vi "Get All Components From Config Browser.vi"() -> (2 "UniqueIDs":string[](array[string]), 3 "Names":string[](array[string]), 5 "error out":errorcluster)   [LabVIEW 2009]
doc: "Gets a list of all configured Horiba Jobin Yvon devices from the computer's registry"
panel:
  in  "error in (no error)":errorcluster
  in  "Config Browser":refnum<k7>
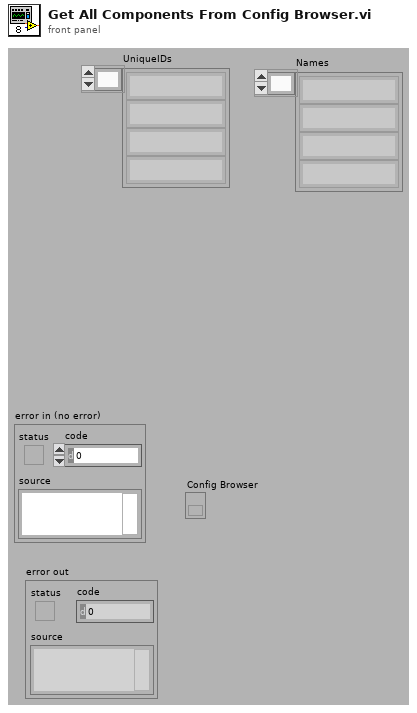
[diagram p1: front panel]
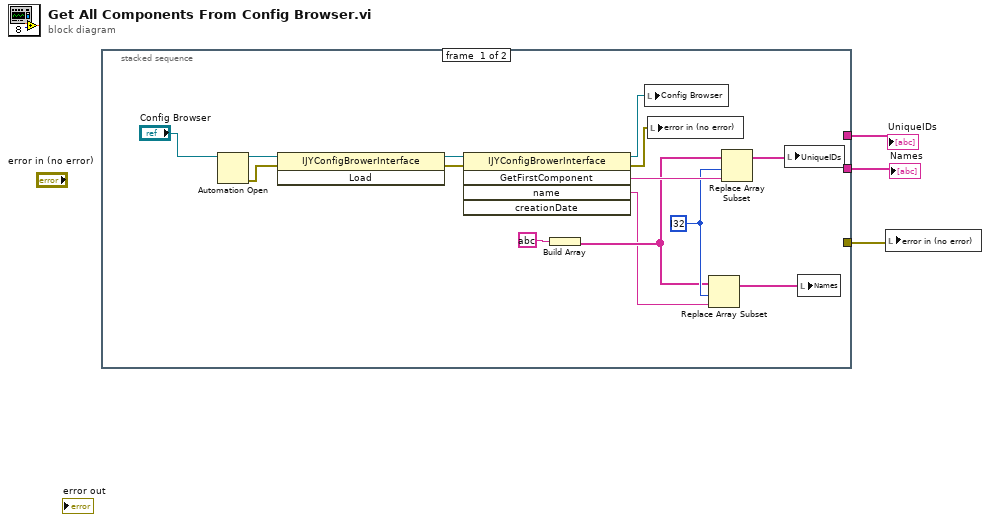
[diagram p0: block diagram]
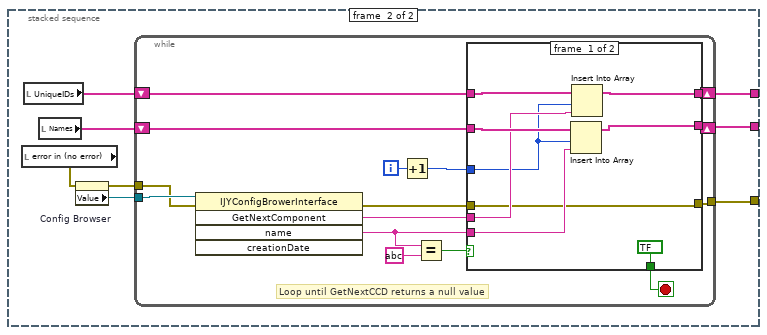
[diagram p2: hidden frame]
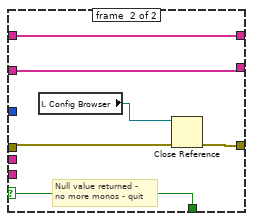
[diagram p3: hidden frame]
diagram:
  n1 = stacked-sequence {
    tunnel: [_ w20] -> w3
    tunnel: [_ w19] -> w2
    tunnel: [_ w18] -> w1
    frame #0 {
      w8 = i32 ?
      n2 = Automation Open(Automation Refnum="Config Browser") -> (Automation Refnum=w17:refnum<k7>, error out=w15:errorcluster)  [unwired: 1 in, 2 out]
      n3 = invoke class="IJYConfigBrowerInterface" method="Load"(reference=w17, error in=w15) -> (reference out=w16:refnum<k7>, error out=w14:errorcluster)  [unwired: 1 in, 1 out]
      n4 = invoke class="IJYConfigBrowerInterface" method="GetFirstComponent"(reference=w16, error in=w14) -> (reference out=w12:refnum<k7>, error out=w10:errorcluster, "GetFirstComponent"=w9:string, "name"=w6:string)  [unwired: 3 in, 1 out]
      n5 = Build Array(string ?) -> (w7:string[])
      n6 = local write "Config Browser"(w12) -> ()
      n7 = local write "error in (no error)"(w10) -> ()
      n8 = Replace Array Subset(array=w7, new element=w6, index=w8) -> (w4:string[])
      n9 = Replace Array Subset(array=w7, new element=w9, index=w8) -> (w5:string[])
      n10 = local write "UniqueIDs"(w5) -> ()
      n11 = local write "Names"(w4) -> ()
    }
    frame #1 {
      n12 = local read "error in (no error)"() -> (w24:errorcluster)
      n13 = local read "UniqueIDs"() -> (w22:string[])
      n14 = local read "Names"() -> (w21:string[])
      n15 = property on="Config Browser" class="Ref (strict)"(error in=w24) -> (error out=w23:errorcluster, "Value"=w25:refnum<k7>)  [unwired: 1 in, 1 out]
      n16 = while {
        tunnel: w25 -> [w40]
        tunnel: w23 -> [w39]
        shift-right: [w26] -> w20
        shift-left: w22 -> [w27]
        shift-right: [w33] -> w19
        shift-left: w21 -> [w34]
        tunnel: [w28] -> w18
        i -> [w38]
        stop <- w35 stop-if-true
        # "Loop until GetNextCCD returns a null value"
        n17 = invoke class="IJYConfigBrowerInterface" method="GetNextComponent"(reference=w40, error in=w39) -> (error out=w29:errorcluster, "GetNextComponent"=w32:string, "name"=w31:string)  [unwired: 3 in, 2 out]
        n18 = Increment(x=w38) -> (x+1=w30:i32)
        n19 = Equal?(x=w31, y=string ?) -> (x = y?=w36:bool)
        n20 = case shown="True" w36 {
          selector: w36 -> [_ w55]
          tunnel: [bool ? w55] -> w35
          tunnel: w27 -> [w42 w54]
          tunnel: w34 -> [w48 w53]
          tunnel: [w44 w53] -> w33
          tunnel: w32 -> [w47 _]
          tunnel: w31 -> [w46 _]
          tunnel: w30 -> [w45 _]
          tunnel: w29 -> [w43 w51]
          tunnel: [w43 w52] -> w28
          tunnel: [w41 w54] -> w26
          frame #0 {
            n21 = Insert Into Array(array=w48, index=w45, new element=w46) -> (w44:string[])
            n22 = Insert Into Array(array=w42, index=w45, new element=w47) -> (w41:string[])
          }
          frame #1 {
            # "Null value returned -\nno more monos - quit"
            n23 = local read "Config Browser"() -> (w50:refnum<k7>)
            n24 = Close Reference(reference=w50, error in (no error)=w51) -> (error out=w52:errorcluster)
          }
        }
      }
    }
  }
  "UniqueIDs" <- w3
  "Names" <- w2
  n25 = local write "error in (no error)"(w1) -> ()
